vi "#632.vi"() -> (3 "Arguments":string)   [LabVIEW 2017, in "testcase-issue.lvclass"]
uses:
  testcase-issue.lvclass
  src/user.lib/_NEVSTOP/Communicable State Machine(CSM)/Utility/_support/Periodic String Filter Level.ctl
  src/user.lib/_NEVSTOP/Communicable State Machine(CSM)/Utility/Periodic String Filter Setting.ctl
  30fe3c43-9356-4971-8d24-89df9aa8dda5.vi
  src/user.lib/_NEVSTOP/Communicable State Machine(CSM)/_Shared/Change Speed Counter.vi
  src/user.lib/_NEVSTOP/Communicable State Machine(CSM)/_Shared/Debounced Signal.vi
  src/user.lib/_NEVSTOP/Communicable State Machine(CSM)/AdvanceAPI/CSM - Revert Arguments-Safe String.vi
  src/user.lib/_NEVSTOP/Communicable State Machine(CSM)/_Shared/Trim Single-line Text.vi
  src/user.lib/_NEVSTOP/Communicable State Machine(CSM)/AdvanceAPI/CSM - Make String Arguments Safe.vi
  src/user.lib/_NEVSTOP/Communicable State Machine(CSM)/AdvanceAPI/CSM - Break Down Multiple States String.vi
  src/user.lib/_NEVSTOP/Communicable State Machine(CSM)/AdvanceAPI/CSM - Compact Multiple States.vi
  src/user.lib/_NEVSTOP/Communicable State Machine(CSM)/AdvanceAPI/CSM - Keywords.vi
  src/user.lib/_NEVSTOP/Communicable State Machine(CSM)/Communicable State Machine.lvlib
  src/user.lib/_NEVSTOP/Communicable State Machine(CSM)/_Shared/CSM Shared.lvlib
panel:
  out "LogInQ":i32
  out "State History":string
  out "log handling Speed(#/s)":dbl
  out "LogInQ change(#/s)":dbl
  out "Level":T1
  in  "Stop":bool
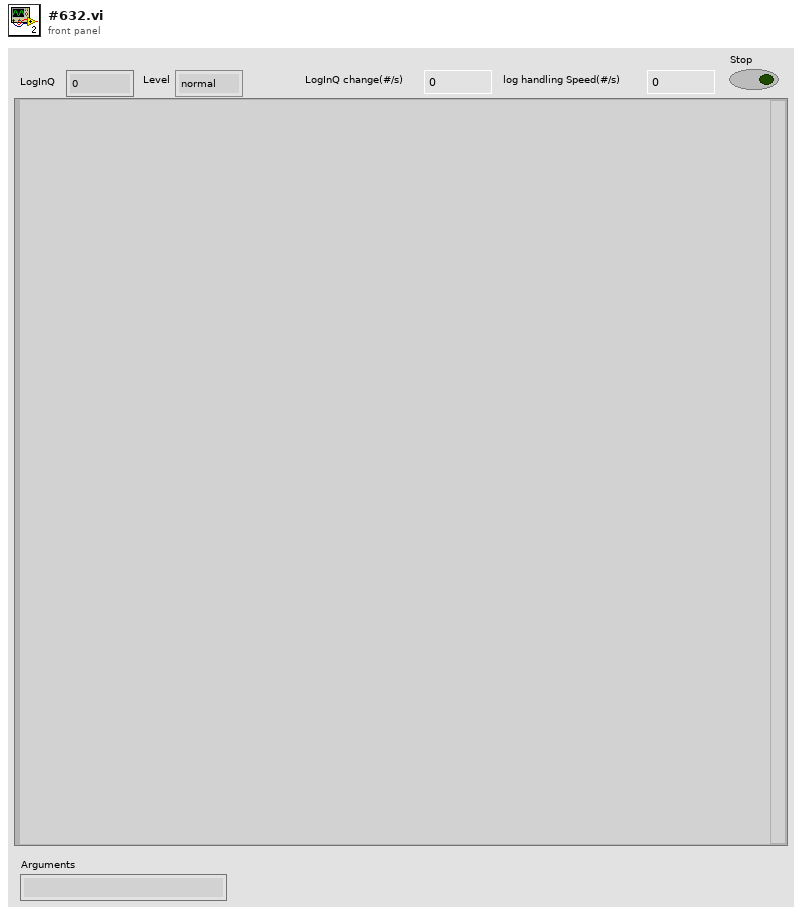
[diagram p1: front panel]
types:
  T1 = typedef "Communicable State Machine.lvlib/Periodic String Filter Level.ctl" = enum16{"normal", "L1", "L2", "L3", "L4"}
  T2 = typedef "Communicable State Machine.lvlib/Periodic String Filter Setting.ctl" = cluster{"threashold(#/s)":dbl, "Check Peroid(s)":dbl}
  T3 = typedef "Communicable State Machine.lvlib/_CSM_GlobalLog_MSG.ctl" = cluster{"Name (\"\" to Use UUID)":string, "Current State":string, "Arguments":string, "Source Message":T4, "Source Module":string, "Complete(T)/Start(F)":bool, "LogType":T5, "Time Stamp":timestamp}
  T4 = typedef "Communicable State Machine.lvlib/_CSM_Response Source Message.ctl" = cluster{"‘State":string, "’Arguments":string, "’Error":errorcluster}
  T5 = typedef "Communicable State Machine.lvlib/_CSM_GlobalLog_MSG_TYPE.ctl" = enum16{"User Log", "State Change", "Status", "Interrupt", "Register", "Unregister", "Error Log", "Module Created", "Module Destroyed", "Async Message", "No-Rep Async Message", "Sync Message", "AsyncMsg Complete", "SyncMsg Complete"}
  T6 = enum32{"Invalid", "Standard", "Closed", "Hidden", "Minimized", "Maximized"}
  T7 = enum32{"invalid app kind", "Development System", "Run Time System", "Student Edition", "Embedded LabVIEW", "Evaluation", "Custom"}
  T8 = cluster{"Current VI Reference":refnum<vi>, "Close Panel on Exit?":bool}
  T9 = cluster{"Core":cluster{"Current VI Reference":refnum<vi>, "Close Panel on Exit?":bool}, "Your Boolean data":bool, "Your string data":string}
  T10 = cluster{"Core":cluster{"Current VI Reference":refnum<vi>, "Close Panel on Exit?":bool}}
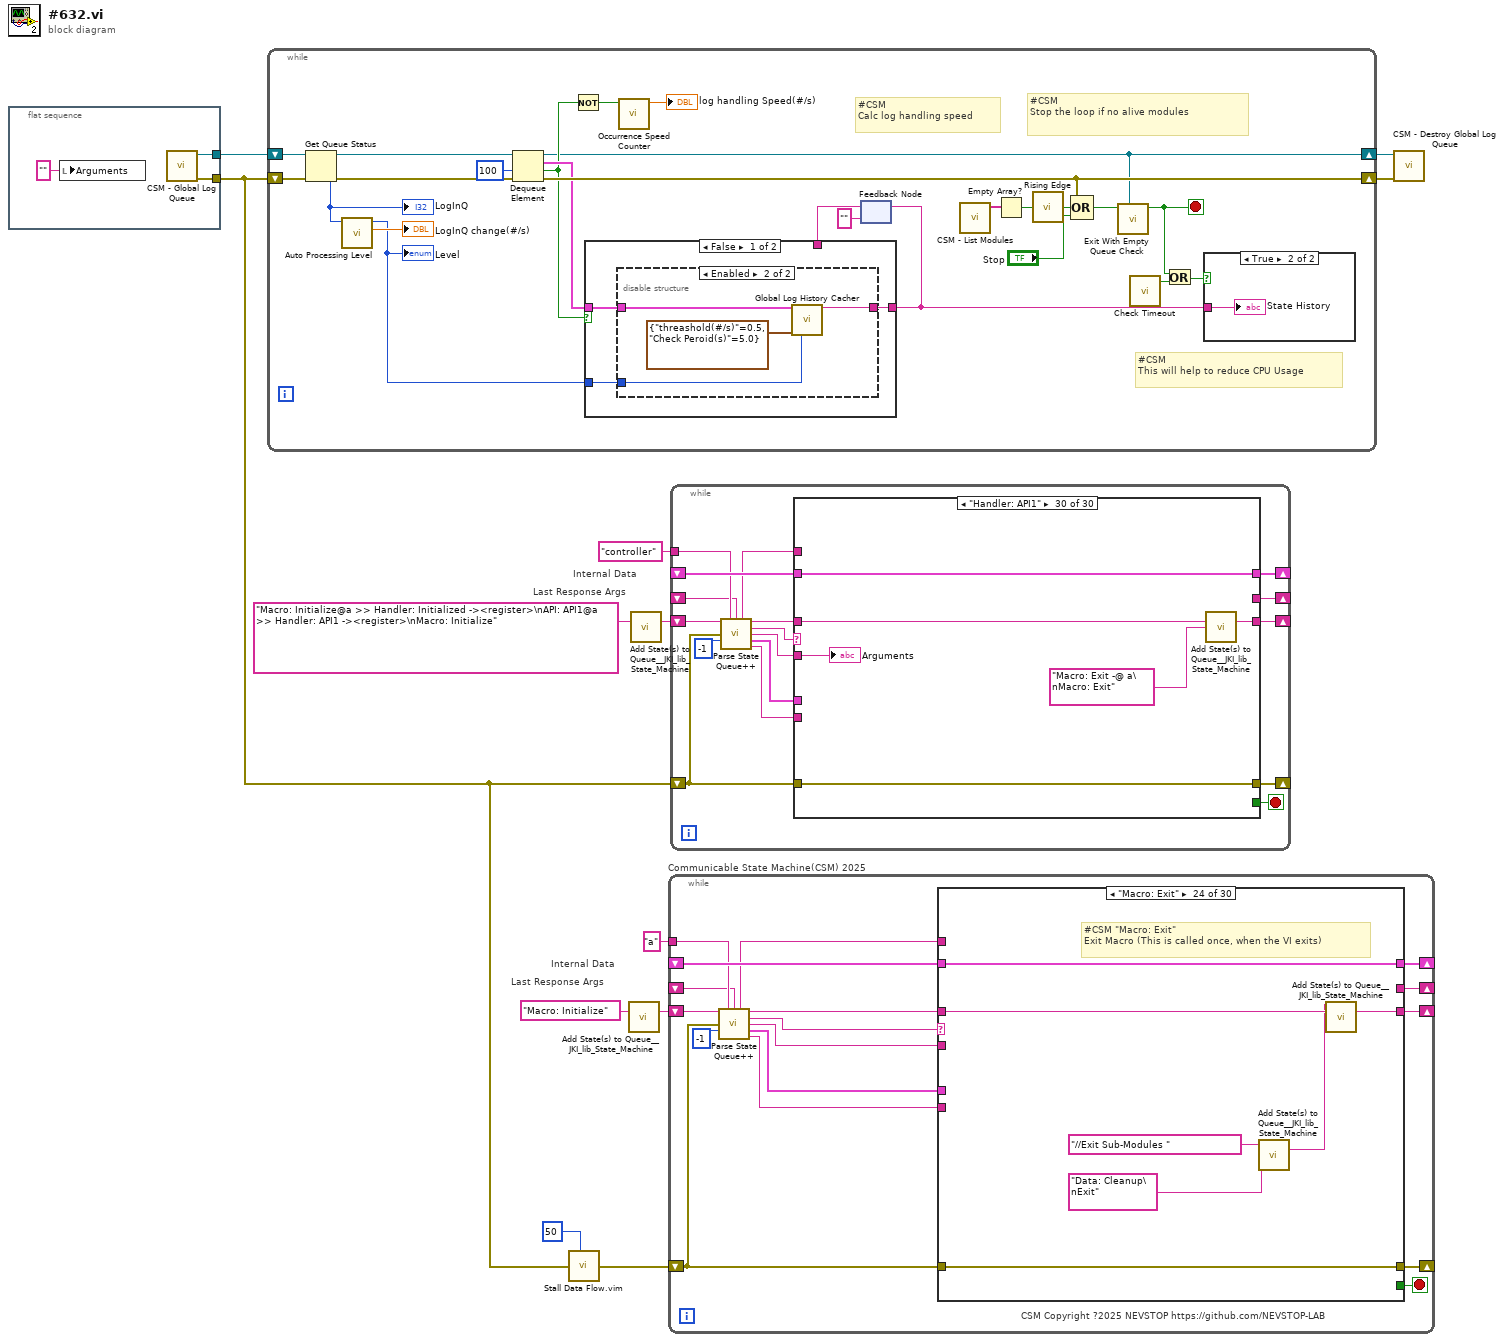
[diagram p0: block diagram]
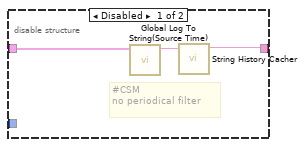
[diagram p2: hidden frame]
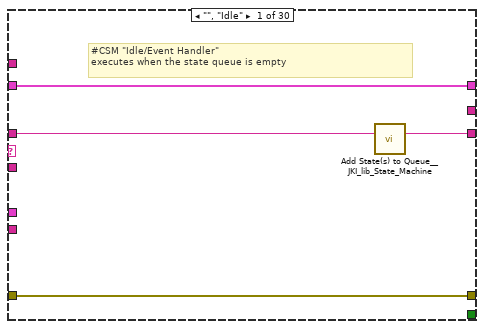
[diagram p5: hidden frame]
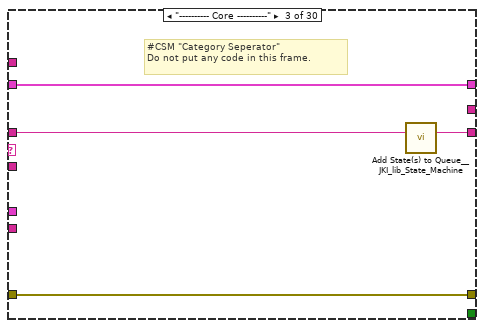
[diagram p7: hidden frame]
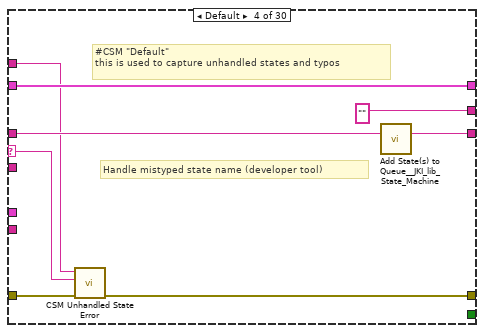
[diagram p8: hidden frame]
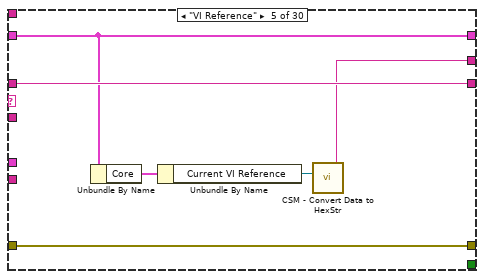
[diagram p9: hidden frame]
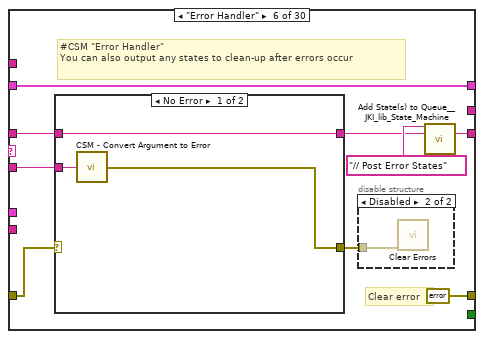
[diagram p10: hidden frame]
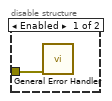
[diagram p11: hidden frame]
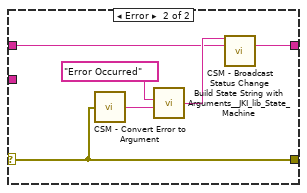
[diagram p12: hidden frame]
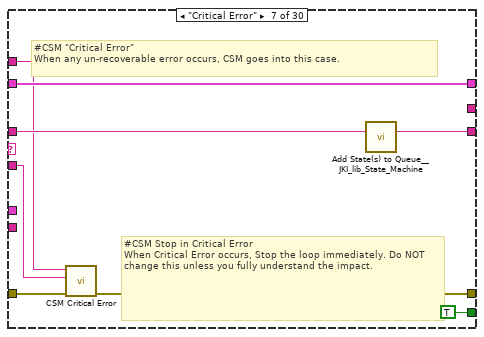
[diagram p13: hidden frame]
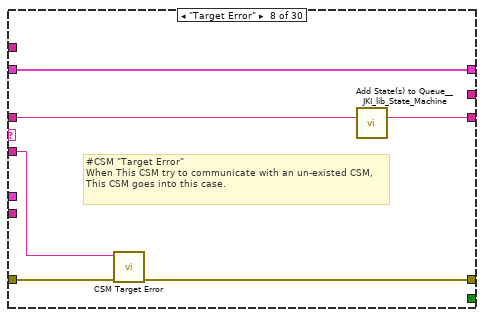
[diagram p14: hidden frame]
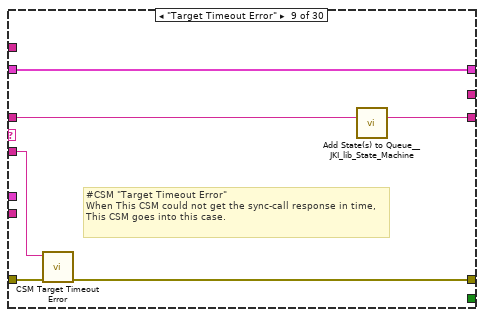
[diagram p15: hidden frame]
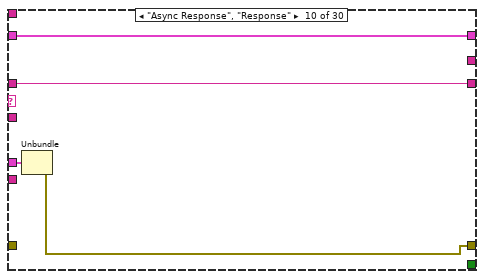
[diagram p16: hidden frame]
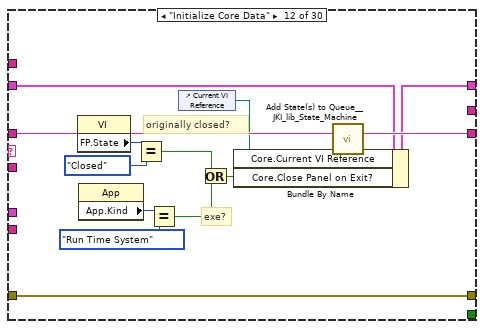
[diagram p18: hidden frame]
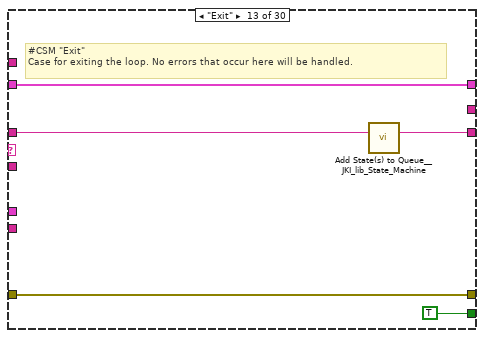
[diagram p19: hidden frame]
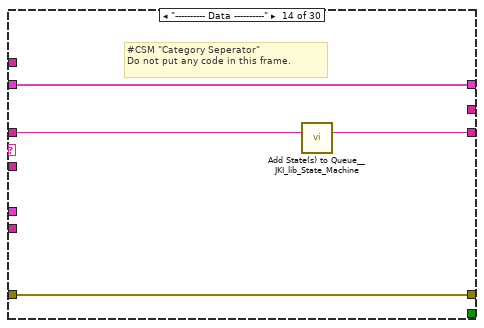
[diagram p20: hidden frame]
diagram:
  # "Last Response Args"
  # "Internal Data"
  # "Last Response Args"
  # "Internal Data"
  n1 = flat-sequence {
    tunnel: [w15] -> w4
    tunnel: [w14] -> w3
    frame #0 {
      n2 = local write "Arguments"("" ("Arguments")) -> ()
      n3 = call "CSM - Global Log Queue.vi"() -> ("error out"=w14:errorcluster, "Global Log Queue"=w15:refnum<queue>)  [unwired: 10 in]
    }
  }
  n4 = while {
    shift-right: [w39] -> w6
    shift-left: w3 -> [w36]
    shift-right: [w23] -> w5
    shift-left: w4 -> [w40]
    stop <- w16 stop-if-true
    # "#CSM\nCalc log handling speed"
    # "#CSM\nStop the loop if no alive modules"
    # "#CSM\nThis will help to reduce CPU Usage"
    n5 = Get Queue Status(queue=w40, error in (no error)=w36) -> (queue out=w38:refnum<queue>, error out=w37:errorcluster, # elements in queue=w19:i32)  [unwired: 1 in, 5 out]
    "LogInQ" <- w19
    n6 = call "Auto Processing Level.vi"("#Left In Q"=w19) -> ("LogInQ Changing Speed (#/s)"=→"LogInQ change(#/s)":dbl, "Level"=w18:T1)  [unwired: 8 in, 1 out]
    "Level" <- w18
    n7 = Dequeue Element(queue=w38, timeout in ms (-1)=100, error in (no error)=w37) -> (queue out=w23:refnum<queue>, element=w35:T3, timed out?=w25:bool, error out=w39:errorcluster)
    n8 = Not(x=w25) -> (.not. x?=w24:bool)
    n9 = call "Occurrence Speed Counter.vi"("Occured? (T)"=w24) -> ("Speed (#/s)"=→"log handling Speed(#/s)":dbl)  [unwired: 8 in, 2 out]
    n10 = feedback #1("" ("String Cache")) -> (w31:string)
    n11 = case shown="False" w25 {
      tunnel: w35 -> [w43 _]
      tunnel: [w42 w51] -> w32
      tunnel: w31 -> [_ w51]
      tunnel: w18 -> [w41 _]
      frame False {
        n12 = disable-structure shown="Enabled" {
          disable-tunnel: w43 -> [w46 w49]
          disable-tunnel: [w44 w50] -> w42
          disable-tunnel: w41 -> [_ w48]
          frame Disabled {
            # "#CSM \nno periodical filter"
            n13 = call "Global Log To String(Source Time).vi"("Log"=w46) -> ("Log String"=w45:string)  [unwired: 9 in]
            n14 = call "String History Cacher.vi"("String"=w45) -> ("String Cache"=w44:string)  [unwired: 10 in]
          }
          frame Enabled {
            n15 = call "Global Log History Cacher.vi"("Global Log Data"=w49, "Settings"=T2 {"threashold(#/s)"=0.5, "Check Peroid(s)"=5.0}, "Level (Normal)"=w48) -> ("String Cache"=w50:string)  [unwired: 12 in]
          }
        }
      }
      frame True {
      }
    }
    n16 = feedback-in #1(w32) -> ()
    n17 = call "CSM - List Modules.vi"() -> ("Module Names"=w30:string[])  [unwired: 10 in, 1 out]
    n18 = Empty Array?(array=w30) -> (empty?=w29:bool)
    n19 = call "Rising Edge.vi"("Signal"=w29) -> ("Rising Edge"=w28:bool)
    n20 = Compound Arithmetic op=OR(w39, w28, "Stop") -> (w21:bool)
    n21 = call "Exit With Empty Queue Check.vi"("Queue"=w23, "Stop"=w21) -> ("Exit"=w16:bool)  [unwired: 8 in, 1 out]
    n22 = call "Check Timeout.vi"() -> ("Timeout"=w33:bool)  [unwired: 8 in]
    n23 = Or(x=w16, y=w33) -> (x .or. y?=w22:bool)
    n24 = case shown="True" w22 {
      tunnel: w32 -> [_ w52]
      frame False {
      }
      frame True {
        "State History" <- w52
      }
    }
  }
  n25 = call "Stall Data Flow.vim"("value in"=w3, "milliseconds to wait"=u32 50) -> ("value out"=w2:errorcluster)  [unwired: 1 out]
  n26 = call <vilib>:"Add State(s) to Queue__JKI_lib_State_Machine.vi"("State(s) in (\"\")"="Macro: Initialize" ("Init State(\"Macro: Initialize\")")) -> ("States Out"=w10:string)  [unwired: 14 in]
  n27 = call <vilib>:"Add State(s) to Queue__JKI_lib_State_Machine.vi"("State(s) in (\"\")"="Macro: Initialize@a >> Handler: Initialized -><register>\nAPI: API1@a >> Handler: API1 -><register>\nMacro: Initialize" ("Init State(\"Macro: Initialize\")")) -> ("States Out"=w9:string)  [unwired: 14 in]
  n28 = while "Communicable State Machine(CSM) 2025" {
    shift-right: [w64] -> _
    shift-left: _ -> [w63]
    shift-right: [w67] -> _
    shift-left: w2 -> [w62]
    shift-right: [w66] -> _
    shift-left: w10 -> [w68]
    tunnel: "a" ("Name (\"\" to Use UUID)") -> [w60]
    shift-right: [w61] -> _
    shift-left: _ -> [w54]
    stop <- w65 stop-if-true
    # "CSM Copyright ?2025 NEVSTOP https://github.com/NEVSTOP-LAB"
    n29 = call "Parse State Queue++.vi"("State Queue"=w68, "Name (\"\" to Use UUID)"=w60, "Response Arguments"=w54, "Previous Error"=w62, "Dequeue (1 ms)"=-1 ("Timeout")) -> ("Name Used"=w55:string, "Remaining States"=w69:string, "Current State"=w59:string, "Arguments"=w58:string, "Additional Information"=w57:T4, "Source CSM"=w56:string)  [unwired: 5 in]
    n30 = case shown="\"Macro: Exit\"" w59 {
      selector: w59 -> [_ _ _ w83 _ _ _ _ _ _ _ _ _ _ _ _ _ _ _ _ _ _ _ _ _ _ _ _ _ _]
      tunnel: w69 -> [w70 w75 w80 w87 w93 w99 w120 w126 w132 w140 w151 w165 w170 w174 w181 w183 w190 w194 w198 w204 w219 w288 w294 w301 w303 w308 w312 w317 w321 w325]
      tunnel: w58 -> [_ _ _ _ _ w98 w116 w125 w130 w139 _ _ _ _ _ _ _ _ _ w199 w213 _ _ _ _ _ _ _ _ _]
      tunnel: w63 -> [w71 w74 w77 w85 w92 w102 w121 w127 w133 w142 w150 w158 w168 w171 _ w182 w185 w191 w196 w202 w215 w285 w291 w298 w302 w307 w311 w314 w318 w322]
      tunnel: [w72 w76 w78 w81 w94 errorcluster {"status"=FALSE, "code"=0, "source"=""} ("error out") w117 w123 w129 w145 w152 w162 w167 w172 w178 w184 w186 w192 w195 w200 w216 w286 w292 w299 w304 w309 w313 w315 w319 w323] -> w67
      tunnel: w62 -> [w72 w76 w78 w88 w94 w100 w122 w124 w131 _ w152 w162 w167 w172 w178 w184 w187 w192 w195 w201 w217 w286 w292 w299 w304 w309 w313 w315 w319 w323]
      tunnel: [w73 w75 w79 w86 w93 w95 w119 w128 w134 w141 w151 w164 w169 w173 w180 w183 w189 w193 w197 w203 w218 w287 w293 w300 w303 w308 w312 w316 w320 w324] -> w66
      tunnel: [_ _ _ _ _ _ TRUE _ _ _ _ _ TRUE _ _ _ _ _ _ _ _ _ _ _ _ _ _ _ _ _] -> w65
      tunnel: [w71 w74 w77 w85 w92 w102 w121 w127 w133 w143 w150 w163 w168 w171 w179 w182 w185 w191 w196 w202 w215 w285 w291 w298 w302 w307 w311 w314 w318 w322] -> w64
      tunnel: w56 -> [_ _ _ _ _ _ _ _ _ w137 _ _ _ _ _ _ _ _ _ _ _ _ _ _ _ _ _ _ _ _]
      tunnel: w57 -> [_ _ _ _ _ _ _ _ _ w144 _ _ _ _ _ _ _ _ _ _ _ _ _ _ _ _ _ _ _ _]
      tunnel: [_ _ _ "" w89 _ _ _ _ _ _ _ _ _ _ _ _ _ _ _ _ _ _ _ _ "Right" "Wrong" ("HEX String (0-9,A-F)") _ _ _] -> w61
      tunnel: w55 -> [_ _ _ w82 _ _ w115 _ _ _ _ _ _ _ _ _ _ _ _ _ _ _ _ _ _ _ _ _ _ _]
      frame "", "Idle" {
        # "#CSM \"Idle/Event Handler\"\nexecutes when the state queue is empty"
        n31 = call <vilib>:"Add State(s) to Queue__JKI_lib_State_Machine.vi"("State(s) in (\"\")"=w70) -> ("States Out"=w73:string)  [unwired: 14 in]
      }
      frame "CSM Documentation" {
        # "#CSM README FIRST\n\nCommunicable State Machine(CSM) is a LabVIEW application framework that builds upon JKI State Machine(JKISM). It follows the pattern of JKISM and extends the keywords to describe message communication between modules, including concepts such as Sync-Message, Async-Message, Subscription/Unsubscription of status - essential elements for creating reusable code modules. For more information, please visit the CSM wiki: https://nevstop-lab.github.io/CSM-Wiki/\n\nFor instructions on JKI State Machine, visit: http://jki.net/state-machine/\nFor information about CSM, visit: https://github.com/NEVSTOP-LAB"
        # "#CSM \"Documentation\"\nCase for holding CSM Documenation"
      }
      frame "---------- Core ----------" {
        # "#CSM \"Category Seperator\"\nDo not put any code in this frame."
        n32 = call <vilib>:"Add State(s) to Queue__JKI_lib_State_Machine.vi"("State(s) in (\"\")"=w80) -> ("States Out"=w79:string)  [unwired: 14 in]
      }
      frame Default {
        # "#CSM \"Default\"\nthis is used to capture unhandled states and typos"
        # "Handle mistyped state name (developer tool)"
        n33 = call "CSM Unhandled State Error.vi"("error in (no error)"=w88, "Undefined State"=w83, "CSM Name"=w82) -> ("error out"=w81:errorcluster)  [unwired: 8 in]
        n34 = call <vilib>:"Add State(s) to Queue__JKI_lib_State_Machine.vi"("State(s) in (\"\")"=w87) -> ("States Out"=w86:string)  [unwired: 14 in]
      }
      frame "VI Reference" {
        n35 = Unbundle By Name(w92) -> ("Core"=w91:T8)
        n36 = Unbundle By Name(w91) -> ("Current VI Reference"=w90:refnum<vi>)
        n37 = call "CSM - Convert Data to HexStr.vi"("Variant"=w90) -> ("HEX String (0-9,A-F)"=w89:string)  [unwired: 8 in]
      }
      frame "Error Handler" {
        # "#CSM Disable this error dialog if you need"
        # "#CSM \"Error Handler\"\nYou can also output any states to clean-up after errors occur"
        # "Clear error"
        n38 = case shown="No Error" w100 {
          selector: w100 -> [_ w109]
          tunnel: [w108 w111] -> w96
          tunnel: w99 -> [w108 w110]
          tunnel: w98 -> [w107 _]
          tunnel: [w106 w109] -> w101
          frame No Error {
            n39 = call "CSM - Convert Argument to Error.vi"("Argument"=w107) -> ("Error"=w106:errorcluster)  [unwired: 4 in]
            n40 = flat-sequence {
              frame #0 {
                # "#CSM External Error Handler Case\nUsually, it's because This CSM register others' \"Error Occurred\" status with \"Error Handler\". If other CSM have any error, the error will be passed here for central handling."
              }
            }
          }
          frame Error {
            # "#CSM Internal Error Handler Case \nIf any error Occurred, \"Error Occurred\" \nstatus update will be broadcasted to system.\nParameter is Error Cluster."
            n41 = call "CSM - Convert Error to Argument.vi"("Error"=w109) -> ("Argument"=w113:string)  [unwired: 4 in]
            n42 = call <vilib>:"Build State String with Arguments__JKI_lib_State_Machine.vi"("Arguments (\"\")"=w113, "State"="Error Occurred" ("Status with Arguments")) -> ("State with Arguments"=w112:string)  [unwired: 4 in]
            n43 = call "CSM - Broadcast Status Change.vi"("Status With Arguments"=w112, "State Queue"=w110) -> ("Remaining States"=w111:string)  [unwired: 13 in]
          }
        }
        n44 = disable-structure shown="Disabled" {
          disable-tunnel: w101 -> [w104 w105]
          frame Enabled {
            n45 = call <vilib>:"General Error Handler.vi"("error in (no error)"=w104) -> ()  [unwired: 10 in, 5 out]
          }
          frame Disabled {
            n46 = call <vilib>:"Clear Errors.vi"("error in (no error)"=w105) -> ()  [unwired: 5 in, 2 out]
          }
        }
        n47 = call <vilib>:"Add State(s) to Queue__JKI_lib_State_Machine.vi"("State(s) in Front (\"\")"="// Post Error States", "State(s) in (\"\")"=w96) -> ("States Out"=w95:string)  [unwired: 13 in]
      }
      frame "Critical Error" {
        # "#CSM Stop in Critical Error\nWhen Critical Error occurs, Stop the loop immediately. Do NOT change this unless you fully understand the impact."
        # "#CSM \"Critical Error\"\nWhen any un-recoverable error occurs, CSM goes into this case."
        n48 = call "CSM Critical Error.vi"("error in (no error)"=w122, "Arugments (As Reason)"=w116, "CSM Name"=w115) -> ("error out"=w117:errorcluster)  [unwired: 8 in]
        n49 = call <vilib>:"Add State(s) to Queue__JKI_lib_State_Machine.vi"("State(s) in (\"\")"=w120) -> ("States Out"=w119:string)  [unwired: 14 in]
      }
      frame "Target Error" {
        # "#CSM \"Target Error\"\nWhen This CSM try to communicate with an un-existed CSM, This CSM goes into this case."
        n50 = call "CSM Target Error.vi"("error in (no error)"=w124, "Arguments (As CSM Name)"=w125) -> ("error out"=w123:errorcluster)  [unwired: 9 in]
        n51 = call <vilib>:"Add State(s) to Queue__JKI_lib_State_Machine.vi"("State(s) in (\"\")"=w126) -> ("States Out"=w128:string)  [unwired: 14 in]
      }
      frame "Target Timeout Error" {
        # "#CSM \"Target Timeout Error\"\nWhen This CSM could not get the sync-call response in time, This CSM goes into this case."
        n52 = call "CSM Target Timeout Error.vi"("error in (no error)"=w131, "Arguments (As CSM Name)"=w130) -> ("error out"=w129:errorcluster)  [unwired: 9 in]
        n53 = call <vilib>:"Add State(s) to Queue__JKI_lib_State_Machine.vi"("State(s) in (\"\")"=w132) -> ("States Out"=w134:string)  [unwired: 14 in]
      }
      frame "Async Response", "Response" {
        n54 = Unbundle(w144) -> ("‘State"=w138:string, "’Arguments"=w136:string, "’Error"=w135:errorcluster)
        n55 = case shown="Default" w138 {
          tunnel: [w149] -> w145
          tunnel: w135 -> [w149]
          tunnel: [w148] -> w143
          tunnel: w142 -> [w148]
          tunnel: [w146] -> w141
          tunnel: w140 -> [w147]
          tunnel: w139 -> [_]
          tunnel: w137 -> [_]
          tunnel: w136 -> [_]
          frame Default {
            # "#CSM Response Comments\nAfter Message is executed, CSM goes to this state for receive the response.\n    For Async Message(->), \"Async Response\" is used. This CSM will goes to \"Async Message Posted\" immediately and receive the \"Async Response\" after the callee finishes the message.\n    For Sync Message(@),  This CSM will wait until the message is done and immediately goes to \"Response\""
            # "#CSM \"Async Response\"\nHandle Async-call Response (\"Async Response\" for ->)"
            # "#CSM \"Response\"\nHandle Sync-call Response (\"Response\" for -@)"
            n56 = call <vilib>:"Add State(s) to Queue__JKI_lib_State_Machine.vi"("State(s) in (\"\")"=w147) -> ("States Out"=w146:string)  [unwired: 14 in]
          }
        }
      }
      frame "Async Message Posted" {
        # "#CSM \"Async Message Posted\"\nAfter Async Message is posted (-> or ->| ), CSM goes to this state for post-action.\nYou can use Argument - State to tell which Async Message is called."
      }
      frame "Initialize Core Data" {
        # "#CSM \"Initialize Core Data\"\nThis is used to determine panel behavior on exit"
        # "originally closed?"
        # "exe?"
        # "If panel starts closed or is an EXE, then close it when we exit"
        n57 = property class="VI"() -> ("FP.State"=w155:T6)  [unwired: 2 in, 2 out]
        n58 = property class="App"() -> ("App.Kind"=w161:T7)  [unwired: 2 in, 2 out]
        n59 = control-ref of="Current VI Reference"() -> (w156:refnum<vi>)
        n60 = Equal?(x=w155, y=T6."Closed" ("Front Panel Window:State")) -> (x = y?=w153:bool)
        n61 = Equal?(x=w161, y=T7."Run Time System" ("Application:Kind")) -> (x = y?=w159:bool)
        n62 = Or(x=w153, y=w159) -> (x .or. y?=w157:bool)
        n63 = Bundle By Name(cluster=w158, "Core.Current VI Reference"=w156, "Core.Close Panel on Exit?"=w157) -> (w163:T9)
        n64 = call <vilib>:"Add State(s) to Queue__JKI_lib_State_Machine.vi"("State(s) in (\"\")"=w165) -> ("States Out"=w164:string)  [unwired: 14 in]
      }
      frame "Exit" {
        # "#CSM \"Exit\"\nCase for exiting the loop. No errors that occur here will be handled."
        n65 = call <vilib>:"Add State(s) to Queue__JKI_lib_State_Machine.vi"("State(s) in (\"\")"=w170) -> ("States Out"=w169:string)  [unwired: 14 in]
      }
      frame "---------- Data ----------" {
        # "#CSM \"Category Seperator\"\nDo not put any code in this frame."
        n66 = call <vilib>:"Add State(s) to Queue__JKI_lib_State_Machine.vi"("State(s) in (\"\")"=w174) -> ("States Out"=w173:string)  [unwired: 14 in]
      }
      frame "Data: Initialize" {
        w175 = T8 {"Current VI Reference"=refnum, "Close Panel on Exit?"=FALSE}  # Core
        w177 = TRUE  # Your Boolean data
        w176 = ""  # Your string data
        # "#CSM do not delete - used by framework"
        # "#CSM Expand Bundle to add new data elements to shift register data."
        # "#CSM Add new data here."
        # "Initialize the shift-register data, here.\n(data names are defined by what you wire into the bundle function)"
        n67 = Bundle("Core"=w175, "Your Boolean data"=w177, "Your string data"=w176) -> (w179:T9)  [unwired: 1 in]
        n68 = call <vilib>:"Add State(s) to Queue__JKI_lib_State_Machine.vi"("State(s) in (\"\")"=w181) -> ("States Out"=w180:string)  [unwired: 14 in]
      }
      frame "Data: Update Indicators" {
      }
      frame "Data: Cleanup" {
        # "Cleanup any data and references, here.\n(this is called automatically, by the Macro: Exit)"
        n69 = Unbundle By Name(w185) -> ("Core.Current VI Reference"=w188:refnum<vi>)
        n70 = Close Reference(reference=w188, error in (no error)=w187) -> (error out=w186:errorcluster)
        n71 = call <vilib>:"Add State(s) to Queue__JKI_lib_State_Machine.vi"("State(s) in (\"\")"=w190) -> ("States Out"=w189:string)  [unwired: 14 in]
      }
      frame "---------- UI ----------" {
        # "#CSM \"Category Seperator\"\nDo not put any code in this frame."
        n72 = call <vilib>:"Add State(s) to Queue__JKI_lib_State_Machine.vi"("State(s) in (\"\")"=w194) -> ("States Out"=w193:string)  [unwired: 14 in]
      }
      frame "UI: Initialize" {
        # "#CSM \"UI: Initialize\"\nInitialize the User Interface, here.\n(this is called automatically, by the Macro: Init)"
        n73 = call <vilib>:"Add State(s) to Queue__JKI_lib_State_Machine.vi"("State(s) in (\"\")"=w198) -> ("States Out"=w197:string)  [unwired: 14 in]
      }
      frame "UI: Cursor Set" {
        # "#CSM \"UI: Cursor Set\"\nSet and Unset Cursor Busy.\n(Usage: \"UI: Cursor Set >> Busy|Idle\")"
        # "Argument"
        n74 = disable-structure shown="TARGET_TYPE!=Windows" {
          disable-tunnel: w201 -> [w207 w212]
          disable-tunnel: [w206 w212] -> w200
          disable-tunnel: w199 -> [w205 _]
          frame condition #0 (active) {
            n75 = case shown="\"Idle\", Default" w205 {
              tunnel: w207 -> [w209 w211]
              tunnel: [w208 w210] -> w206
              frame "Idle", Default {
                n76 = call <vilib>:"Unset Busy.vi"("error in (no error)"=w209) -> ("error out"=w208:errorcluster)  [unwired: 10 in]
              }
              frame "Busy" {
                n77 = call <vilib>:"Set Busy.vi"("error in (no error)"=w211) -> ("error out"=w210:errorcluster)  [unwired: 9 in, 1 out]
              }
            }
          }
          frame condition #1 {
          }
        }
        n78 = call <vilib>:"Add State(s) to Queue__JKI_lib_State_Machine.vi"("State(s) in (\"\")"=w204) -> ("States Out"=w203:string)  [unwired: 14 in]
      }
      frame "UI: Front Panel State" {
        # "#CSM \"UI: Front Panel State\"\nSet Front Panel Open or Closed\n(Usage: \"UI: Front Panel State >> Open|Close\")"
        # "Argument"
        n79 = Unbundle By Name(w215) -> ("Core.Current VI Reference"=w214:refnum<vi>)
        n80 = call <vilib>:"Add State(s) to Queue__JKI_lib_State_Machine.vi"("State(s) in (\"\")"=w219) -> ("States Out"=w218:string)  [unwired: 14 in]
        n81 = case shown="\"Close\", \"Closed\"" w213 {
          tunnel: w217 -> [w225 w240 w251 w264 w277]
          tunnel: [w227 w241 w253 w266 w279] -> w216
          tunnel: w214 -> [w226 w238 w252 w265 w278]
          frame "Open", "Standard", Default {
            w220 = T6."Standard" ("State")
            n82 = property class="VI"(reference=w226, error in=w225) -> (reference out=w223:refnum<vi>, error out=w224:errorcluster, "FP.State"=w222:T6)
            n83 = Not Equal?(x=w222, y=w220) -> (x != y?=w221:bool)
            n84 = case shown="True" w221 {
              tunnel: [w231 w233] -> w227
              tunnel: w224 -> [w230 w233]
              tunnel: w223 -> [w229 _]
              tunnel: w220 -> [w228 _]
              frame True {
                n85 = invoke class="VI" method="FP.Open"(reference=w229, error in=w230, "Activate"=TRUE, "State"=w228) -> (error out=w231:errorcluster)  [unwired: 1 in, 4 out]
              }
              frame False {
              }
            }
          }
          frame "Close", "Closed" {
            n86 = property class="VI"(reference=w238, error in=w240) -> (reference out=w237:refnum<vi>, error out=w239:errorcluster, "FP.State"=w235:T6)
            n87 = Not Equal?(x=w235, y=T6."Closed" ("Front Panel Window:State")) -> (x != y?=w234:bool)
            n88 = case shown="False" w234 {
              tunnel: [w242 w245] -> w241
              tunnel: w239 -> [w242 w244]
              tunnel: w237 -> [_ w243]
              frame False {
              }
              frame True {
                n89 = invoke class="VI" method="FP.Close"(reference=w243, error in=w244) -> (error out=w245:errorcluster)  [unwired: 1 in, 2 out]
              }
            }
          }
          frame "Hidden", "Hide" {
            w246 = T6."Hidden" ("State")
            n90 = property class="VI"(reference=w252, error in=w251) -> (reference out=w249:refnum<vi>, error out=w250:errorcluster, "FP.State"=w248:T6)
            n91 = Not Equal?(x=w248, y=w246) -> (x != y?=w247:bool)
            n92 = case shown="True" w247 {
              tunnel: [w257 w258] -> w253
              tunnel: w250 -> [w256 w258]
              tunnel: w249 -> [w255 _]
              tunnel: w246 -> [w254 _]
              frame True {
                n93 = invoke class="VI" method="FP.Open"(reference=w255, error in=w256, "State"=w254) -> (error out=w257:errorcluster)  [unwired: 2 in, 4 out]
              }
              frame False {
              }
            }
          }
          frame "Minimize", "Minimized" {
            w259 = T6."Minimized" ("State")
            n94 = property class="VI"(reference=w265, error in=w264) -> (reference out=w262:refnum<vi>, error out=w263:errorcluster, "FP.State"=w261:T6)
            n95 = Not Equal?(x=w261, y=w259) -> (x != y?=w260:bool)
            n96 = case shown="True" w260 {
              tunnel: [w270 w271] -> w266
              tunnel: w263 -> [w269 w271]
              tunnel: w262 -> [w268 _]
              tunnel: w259 -> [w267 _]
              frame True {
                n97 = invoke class="VI" method="FP.Open"(reference=w268, error in=w269, "State"=w267) -> (error out=w270:errorcluster)  [unwired: 2 in, 4 out]
              }
              frame False {
              }
            }
          }
          frame "Maximize", "Maximized" {
            w272 = T6."Maximized" ("State")
            n98 = property class="VI"(reference=w278, error in=w277) -> (reference out=w275:refnum<vi>, error out=w276:errorcluster, "FP.State"=w274:T6)
            n99 = Not Equal?(x=w274, y=w272) -> (x != y?=w273:bool)
            n100 = case shown="True" w273 {
              tunnel: [w283 w284] -> w279
              tunnel: w276 -> [w282 w284]
              tunnel: w275 -> [w281 _]
              tunnel: w272 -> [w280 _]
              frame True {
                n101 = invoke class="VI" method="FP.Open"(reference=w281, error in=w282, "State"=w280) -> (error out=w283:errorcluster)  [unwired: 2 in, 4 out]
              }
              frame False {
              }
            }
          }
        }
      }
      frame "---------- Macro ----------" {
        # "#CSM \"Category Seperator\"\nDo not put any code in this frame."
        n102 = call <vilib>:"Add State(s) to Queue__JKI_lib_State_Machine.vi"("State(s) in (\"\")"=w288) -> ("States Out"=w287:string)  [unwired: 14 in]
      }
      frame "Macro: Initialize" {
        # "#CSM \"Macro: Initialize\"\nInitialization Macro (This is called once, when the VI starts)"
        n103 = call <vilib>:"Add State(s) to Queue__JKI_lib_State_Machine.vi"("State(s) in Front (\"\")"="Data: Initialize\nInitialize Core Data\nData: Update Indicators", "State(s) in (\"\")"=w294, "State(s) at Back (\"\")"="API: API1") -> ("States Out"=w293:string)  [unwired: 12 in]
      }
      frame "Macro: Exit" {
        # "#CSM \"Macro: Exit\"\nExit Macro (This is called once, when the VI exits)"
        n104 = call <vilib>:"Add State(s) to Queue__JKI_lib_State_Machine.vi"("State(s) in Front (\"\")"="//Exit Sub-Modules ", "State(s) at Back (\"\")"="Data: Cleanup\nExit") -> ("States Out"=w296:string)  [unwired: 13 in]
        n105 = call <vilib>:"Add State(s) to Queue__JKI_lib_State_Machine.vi"("State(s) in Front (\"\")"=w296, "State(s) in (\"\")"=w301) -> ("States Out"=w300:string)  [unwired: 13 in]
      }
      frame "---------- API ----------" {
        # "#CSM \"Category Seperator\"\nDo not put any code in this frame."
      }
      frame "API: API1" {
        # "#CSM API Example\nCopy/Rename this case for your own API"
        n106 = Wait (ms)(milliseconds to wait=u32 2000) -> ()  [unwired: 1 out]
      }
      frame "API: API2" {
        # "#CSM API Example\nCopy/Rename this case for your own API"
      }
      frame "---------- Action ----------" {
        # "#CSM \"Category Seperator\"\nDo not put any code in this frame."
        n107 = call <vilib>:"Add State(s) to Queue__JKI_lib_State_Machine.vi"("State(s) in (\"\")"=w317) -> ("States Out"=w316:string)  [unwired: 14 in]
      }
      frame "Action: action1" {
        # "#CSM \"Internal State\"\nThis category is used for holding internal states"
        n108 = call <vilib>:"Add State(s) to Queue__JKI_lib_State_Machine.vi"("State(s) in (\"\")"=w321) -> ("States Out"=w320:string)  [unwired: 14 in]
      }
      frame "Action: action2" {
        # "#CSM \"Internal State\"\nThis category is used for holding internal states"
        n109 = call <vilib>:"Add State(s) to Queue__JKI_lib_State_Machine.vi"("State(s) in (\"\")"=w325) -> ("States Out"=w324:string)  [unwired: 14 in]
      }
    }
  }
  n110 = while {
    shift-right: [w337] -> _
    shift-left: _ -> [w336]
    shift-right: [w340] -> _
    shift-left: w3 -> [w335]
    shift-right: [w339] -> _
    shift-left: w9 -> [w341]
    tunnel: "controller" ("Name (\"\" to Use UUID)") -> [w333]
    shift-right: [w334] -> _
    shift-left: _ -> [w327]
    stop <- w338 stop-if-true
    n111 = call "Parse State Queue++.vi"("State Queue"=w341, "Name (\"\" to Use UUID)"=w333, "Response Arguments"=w327, "Previous Error"=w335, "Dequeue (1 ms)"=-1 ("Timeout")) -> ("Name Used"=w328:string, "Remaining States"=w342:string, "Current State"=w332:string, "Arguments"=w331:string, "Additional Information"=w330:T4, "Source CSM"=w329:string)  [unwired: 5 in]
    n112 = case shown="\"Handler: API1\"" w332 {
      selector: w332 -> [_ _ _ w356 _ _ _ _ _ _ _ _ _ _ _ _ _ _ _ _ _ _ _ _ _ _ _ _ _ _]
      tunnel: w342 -> [w343 w348 w353 w360 w366 w372 w393 w399 w405 w409 w413 w427 w432 w436 w441 w443 w450 w454 w458 w464 w479 w548 w553 w560 w562 w567 w571 w576 w583 w589]
      tunnel: w331 -> [_ _ _ _ _ w371 w389 w398 w403 _ _ _ _ _ _ _ _ _ _ w459 w473 _ _ _ _ _ _ _ _ w584]
      tunnel: w336 -> [w344 w347 w350 w358 w365 w375 w394 w400 w406 w410 w412 w420 w430 w433 _ w442 w445 w451 w456 w462 w475 w545 w550 w557 w561 w566 w570 w573 w581 w586]
      tunnel: [w345 w349 w351 w354 w367 errorcluster {"status"=FALSE, "code"=0, "source"=""} ("error out") w390 w396 w402 w408 w414 w424 w429 w434 w438 w444 w446 w452 w455 w460 w476 w546 w551 w558 w563 w568 w572 w574 w578 w587] -> w340
      tunnel: w335 -> [w345 w349 w351 w361 w367 w373 w395 w397 w404 _ w414 w424 w429 w434 w438 w444 w447 w452 w455 w461 w477 w546 w551 w558 w563 w568 w572 w574 _ w587]
      tunnel: [w346 w348 w352 w359 w366 w368 w392 w401 w407 w409 w413 w426 w431 w435 w440 w443 w449 w453 w457 w463 w478 w547 w552 w559 w562 w567 w571 w575 w582 w588] -> w339
      tunnel: [_ _ _ _ _ _ TRUE _ _ _ _ _ TRUE _ _ _ _ _ _ _ _ _ _ _ _ _ _ _ _ _] -> w338
      tunnel: [w344 w347 w350 w358 w365 w375 w394 w400 w406 w410 w412 w425 w430 w433 w439 w442 w445 w451 w456 w462 w475 w545 w550 w557 w561 w566 w570 w573 w581 w586] -> w337
      tunnel: w329 -> [_ _ _ _ _ _ _ _ _ _ _ _ _ _ _ _ _ _ _ _ _ _ _ _ _ _ _ _ _ _]
      tunnel: w330 -> [_ _ _ _ _ _ _ _ _ w411 _ _ _ _ _ _ _ _ _ _ _ _ _ _ _ _ _ _ _ _]
      tunnel: [_ _ _ "" w362 _ _ _ _ _ _ _ _ _ _ _ _ _ _ _ _ _ _ _ _ "Right" "Wrong" ("HEX String (0-9,A-F)") _ _ _] -> w334
      tunnel: w328 -> [_ _ _ w355 _ _ w388 _ _ _ _ _ _ _ _ _ _ _ _ _ _ _ _ _ _ _ _ _ w580 _]
      frame "", "Idle" {
        # "#CSM \"Idle/Event Handler\"\nexecutes when the state queue is empty"
        n113 = call <vilib>:"Add State(s) to Queue__JKI_lib_State_Machine.vi"("State(s) in (\"\")"=w343) -> ("States Out"=w346:string)  [unwired: 14 in]
      }
      frame "CSM Documentation" {
        # "#CSM \"Documentation\"\nCase for holding CSM Documenation"
      }
      frame "---------- Core ----------" {
        # "#CSM \"Category Seperator\"\nDo not put any code in this frame."
        n114 = call <vilib>:"Add State(s) to Queue__JKI_lib_State_Machine.vi"("State(s) in (\"\")"=w353) -> ("States Out"=w352:string)  [unwired: 14 in]
      }
      frame Default {
        # "#CSM \"Default\"\nthis is used to capture unhandled states and typos"
        # "Handle mistyped state name (developer tool)"
        n115 = call "CSM Unhandled State Error.vi"("error in (no error)"=w361, "Undefined State"=w356, "CSM Name"=w355) -> ("error out"=w354:errorcluster)  [unwired: 8 in]
        n116 = call <vilib>:"Add State(s) to Queue__JKI_lib_State_Machine.vi"("State(s) in (\"\")"=w360) -> ("States Out"=w359:string)  [unwired: 14 in]
      }
      frame "VI Reference" {
        n117 = Unbundle By Name(w365) -> ("Core"=w364:T8)
        n118 = Unbundle By Name(w364) -> ("Current VI Reference"=w363:refnum<vi>)
        n119 = call "CSM - Convert Data to HexStr.vi"("Variant"=w363) -> ("HEX String (0-9,A-F)"=w362:string)  [unwired: 8 in]
      }
      frame "Error Handler" {
        # "#CSM \"Error Handler\"\nYou can also output any states to clean-up after errors occur"
        # "Clear error"
        n120 = case shown="No Error" w373 {
          selector: w373 -> [_ w382]
          tunnel: [w381 w384] -> w369
          tunnel: w372 -> [w381 w383]
          tunnel: w371 -> [w380 _]
          tunnel: [w379 w382] -> w374
          frame No Error {
            n121 = call "CSM - Convert Argument to Error.vi"("Argument"=w380) -> ("Error"=w379:errorcluster)  [unwired: 4 in]
          }
          frame Error {
            n122 = call "CSM - Convert Error to Argument.vi"("Error"=w382) -> ("Argument"=w386:string)  [unwired: 4 in]
            n123 = call <vilib>:"Build State String with Arguments__JKI_lib_State_Machine.vi"("Arguments (\"\")"=w386, "State"="Error Occurred" ("Status with Arguments")) -> ("State with Arguments"=w385:string)  [unwired: 4 in]
            n124 = call "CSM - Broadcast Status Change.vi"("Status With Arguments"=w385, "State Queue"=w383) -> ("Remaining States"=w384:string)  [unwired: 13 in]
          }
        }
        n125 = disable-structure shown="Disabled" {
          disable-tunnel: w374 -> [w377 w378]
          frame Enabled {
            n126 = call <vilib>:"General Error Handler.vi"("error in (no error)"=w377) -> ()  [unwired: 10 in, 5 out]
          }
          frame Disabled {
            n127 = call <vilib>:"Clear Errors.vi"("error in (no error)"=w378) -> ()  [unwired: 5 in, 2 out]
          }
        }
        n128 = call <vilib>:"Add State(s) to Queue__JKI_lib_State_Machine.vi"("State(s) in Front (\"\")"="// Post Error States", "State(s) in (\"\")"=w369) -> ("States Out"=w368:string)  [unwired: 13 in]
      }
      frame "Critical Error" {
        # "#CSM Stop in Critical Error\nWhen Critical Error occurs, Stop the loop immediately. Do NOT change this unless you fully understand the impact."
        # "#CSM \"Critical Error\"\nWhen any un-recoverable error occurs, CSM goes into this case."
        n129 = call "CSM Critical Error.vi"("error in (no error)"=w395, "Arugments (As Reason)"=w389, "CSM Name"=w388) -> ("error out"=w390:errorcluster)  [unwired: 8 in]
        n130 = call <vilib>:"Add State(s) to Queue__JKI_lib_State_Machine.vi"("State(s) in (\"\")"=w393) -> ("States Out"=w392:string)  [unwired: 14 in]
      }
      frame "Target Error" {
        # "#CSM \"Target Error\"\nWhen This CSM try to communicate with an un-existed CSM, This CSM goes into this case."
        n131 = call "CSM Target Error.vi"("error in (no error)"=w397, "Arguments (As CSM Name)"=w398) -> ("error out"=w396:errorcluster)  [unwired: 9 in]
        n132 = call <vilib>:"Add State(s) to Queue__JKI_lib_State_Machine.vi"("State(s) in (\"\")"=w399) -> ("States Out"=w401:string)  [unwired: 14 in]
      }
      frame "Target Timeout Error" {
        # "#CSM \"Target Timeout Error\"\nWhen This CSM could not get the sync-call response in time, This CSM goes into this case."
        n133 = call "CSM Target Timeout Error.vi"("error in (no error)"=w404, "Arguments (As CSM Name)"=w403) -> ("error out"=w402:errorcluster)  [unwired: 9 in]
        n134 = call <vilib>:"Add State(s) to Queue__JKI_lib_State_Machine.vi"("State(s) in (\"\")"=w405) -> ("States Out"=w407:string)  [unwired: 14 in]
      }
      frame "Async Response", "Response" {
        n135 = Unbundle(w411) -> ("’Error"=w408:errorcluster)  [unwired: 2 out]
      }
      frame "Async Message Posted" {
        # "#CSM \"Async Message Posted\"\nAfter Async Message is posted (-> or ->| ), CSM goes to this state for post-action.\nYou can use Argument - State to tell which Async Message is called."
      }
      frame "Initialize Core Data" {
        # "originally closed?"
        # "exe?"
        n136 = property class="VI"() -> ("FP.State"=w417:T6)  [unwired: 2 in, 2 out]
        n137 = property class="App"() -> ("App.Kind"=w423:T7)  [unwired: 2 in, 2 out]
        n138 = Equal?(x=w417, y=T6."Closed" ("Front Panel Window:State")) -> (x = y?=w415:bool)
        n139 = Equal?(x=w423, y=T7."Run Time System" ("Application:Kind")) -> (x = y?=w421:bool)
        n140 = control-ref of="Current VI Reference"() -> (w418:refnum<vi>)
        n141 = Or(x=w415, y=w421) -> (x .or. y?=w419:bool)
        n142 = Bundle By Name(cluster=w420, "Core.Current VI Reference"=w418, "Core.Close Panel on Exit?"=w419) -> (w425:T10)
        n143 = call <vilib>:"Add State(s) to Queue__JKI_lib_State_Machine.vi"("State(s) in (\"\")"=w427) -> ("States Out"=w426:string)  [unwired: 14 in]
      }
      frame "Exit" {
        # "#CSM \"Exit\"\nCase for exiting the loop. No errors that occur here will be handled."
        n144 = call <vilib>:"Add State(s) to Queue__JKI_lib_State_Machine.vi"("State(s) in (\"\")"=w432) -> ("States Out"=w431:string)  [unwired: 14 in]
      }
      frame "---------- Data ----------" {
        # "#CSM \"Category Seperator\"\nDo not put any code in this frame."
        n145 = call <vilib>:"Add State(s) to Queue__JKI_lib_State_Machine.vi"("State(s) in (\"\")"=w436) -> ("States Out"=w435:string)  [unwired: 14 in]
      }
      frame "Data: Initialize" {
        w437 = T8 {"Current VI Reference"=refnum, "Close Panel on Exit?"=FALSE}  # Core
        # "Initialize the shift-register data, here.\n(data names are defined by what you wire into the bundle function)"
        n146 = Bundle("Core"=w437) -> (w439:T10)  [unwired: 1 in]
        n147 = call <vilib>:"Add State(s) to Queue__JKI_lib_State_Machine.vi"("State(s) in (\"\")"=w441) -> ("States Out"=w440:string)  [unwired: 14 in]
      }
      frame "Data: Update Indicators" {
      }
      frame "Data: Cleanup" {
        # "Cleanup any data and references, here.\n(this is called automatically, by the Macro: Exit)"
        n148 = Unbundle By Name(w445) -> ("Core.Current VI Reference"=w448:refnum<vi>)
        n149 = Close Reference(reference=w448, error in (no error)=w447) -> (error out=w446:errorcluster)
        n150 = call <vilib>:"Add State(s) to Queue__JKI_lib_State_Machine.vi"("State(s) in (\"\")"=w450) -> ("States Out"=w449:string)  [unwired: 14 in]
      }
      frame "---------- UI ----------" {
        # "#CSM \"Category Seperator\"\nDo not put any code in this frame."
        n151 = call <vilib>:"Add State(s) to Queue__JKI_lib_State_Machine.vi"("State(s) in (\"\")"=w454) -> ("States Out"=w453:string)  [unwired: 14 in]
      }
      frame "UI: Initialize" {
        # "#CSM \"UI: Initialize\"\nInitialize the User Interface, here.\n(this is called automatically, by the Macro: Init)"
        n152 = call <vilib>:"Add State(s) to Queue__JKI_lib_State_Machine.vi"("State(s) in (\"\")"=w458) -> ("States Out"=w457:string)  [unwired: 14 in]
      }
      frame "UI: Cursor Set" {
        # "#CSM \"UI: Cursor Set\"\nSet and Unset Cursor Busy.\n(Usage: \"UI: Cursor Set >> Busy|Idle\")"
        # "Argument"
        n153 = disable-structure shown="Default" {
          disable-tunnel: w461 -> [w467 w472]
          disable-tunnel: [w466 w472] -> w460
          disable-tunnel: w459 -> [w465 _]
          frame condition #0 (active) {
            n154 = case shown="\"Idle\", Default" w465 {
              tunnel: w467 -> [w469 w471]
              tunnel: [w468 w470] -> w466
              frame "Idle", Default {
                n155 = call <vilib>:"Unset Busy.vi"("error in (no error)"=w469) -> ("error out"=w468:errorcluster)  [unwired: 10 in]
              }
              frame "Busy" {
                n156 = call <vilib>:"Set Busy.vi"("error in (no error)"=w471) -> ("error out"=w470:errorcluster)  [unwired: 9 in, 1 out]
              }
            }
          }
          frame condition #1 {
          }
        }
        n157 = call <vilib>:"Add State(s) to Queue__JKI_lib_State_Machine.vi"("State(s) in (\"\")"=w464) -> ("States Out"=w463:string)  [unwired: 14 in]
      }
      frame "UI: Front Panel State" {
        # "#CSM \"UI: Front Panel State\"\nSet Front Panel Open or Closed\n(Usage: \"UI: Front Panel State >> Open|Close\")"
        # "Argument"
        n158 = Unbundle By Name(w475) -> ("Core.Current VI Reference"=w474:refnum<vi>)
        n159 = call <vilib>:"Add State(s) to Queue__JKI_lib_State_Machine.vi"("State(s) in (\"\")"=w479) -> ("States Out"=w478:string)  [unwired: 14 in]
        n160 = case shown="\"Close\", \"Closed\"" w473 {
          tunnel: w477 -> [w485 w500 w511 w524 w537]
          tunnel: [w487 w501 w513 w526 w539] -> w476
          tunnel: w474 -> [w486 w498 w512 w525 w538]
          frame "Open", "Standard", Default {
            w480 = T6."Standard" ("State")
            n161 = property class="VI"(reference=w486, error in=w485) -> (reference out=w483:refnum<vi>, error out=w484:errorcluster, "FP.State"=w482:T6)
            n162 = Not Equal?(x=w482, y=w480) -> (x != y?=w481:bool)
            n163 = case shown="True" w481 {
              tunnel: [w491 w493] -> w487
              tunnel: w484 -> [w490 w493]
              tunnel: w483 -> [w489 _]
              tunnel: w480 -> [w488 _]
              frame True {
                n164 = invoke class="VI" method="FP.Open"(reference=w489, error in=w490, "Activate"=TRUE, "State"=w488) -> (error out=w491:errorcluster)  [unwired: 1 in, 4 out]
              }
              frame False {
              }
            }
          }
          frame "Close", "Closed" {
            n165 = property class="VI"(reference=w498, error in=w500) -> (reference out=w497:refnum<vi>, error out=w499:errorcluster, "FP.State"=w495:T6)
            n166 = Not Equal?(x=w495, y=T6."Closed" ("Front Panel Window:State")) -> (x != y?=w494:bool)
            n167 = case shown="False" w494 {
              tunnel: [w502 w505] -> w501
              tunnel: w499 -> [w502 w504]
              tunnel: w497 -> [_ w503]
              frame False {
              }
              frame True {
                n168 = invoke class="VI" method="FP.Close"(reference=w503, error in=w504) -> (error out=w505:errorcluster)  [unwired: 1 in, 2 out]
              }
            }
          }
          frame "Hidden", "Hide" {
            w506 = T6."Hidden" ("State")
            n169 = property class="VI"(reference=w512, error in=w511) -> (reference out=w509:refnum<vi>, error out=w510:errorcluster, "FP.State"=w508:T6)
            n170 = Not Equal?(x=w508, y=w506) -> (x != y?=w507:bool)
            n171 = case shown="True" w507 {
              tunnel: [w517 w518] -> w513
              tunnel: w510 -> [w516 w518]
              tunnel: w509 -> [w515 _]
              tunnel: w506 -> [w514 _]
              frame True {
                n172 = invoke class="VI" method="FP.Open"(reference=w515, error in=w516, "State"=w514) -> (error out=w517:errorcluster)  [unwired: 2 in, 4 out]
              }
              frame False {
              }
            }
          }
          frame "Minimize", "Minimized" {
            w519 = T6."Minimized" ("State")
            n173 = property class="VI"(reference=w525, error in=w524) -> (reference out=w522:refnum<vi>, error out=w523:errorcluster, "FP.State"=w521:T6)
            n174 = Not Equal?(x=w521, y=w519) -> (x != y?=w520:bool)
            n175 = case shown="True" w520 {
              tunnel: [w530 w531] -> w526
              tunnel: w523 -> [w529 w531]
              tunnel: w522 -> [w528 _]
              tunnel: w519 -> [w527 _]
              frame True {
                n176 = invoke class="VI" method="FP.Open"(reference=w528, error in=w529, "State"=w527) -> (error out=w530:errorcluster)  [unwired: 2 in, 4 out]
              }
              frame False {
              }
            }
          }
          frame "Maximize", "Maximized" {
            w532 = T6."Maximized" ("State")
            n177 = property class="VI"(reference=w538, error in=w537) -> (reference out=w535:refnum<vi>, error out=w536:errorcluster, "FP.State"=w534:T6)
            n178 = Not Equal?(x=w534, y=w532) -> (x != y?=w533:bool)
            n179 = case shown="True" w533 {
              tunnel: [w543 w544] -> w539
              tunnel: w536 -> [w542 w544]
              tunnel: w535 -> [w541 _]
              tunnel: w532 -> [w540 _]
              frame True {
                n180 = invoke class="VI" method="FP.Open"(reference=w541, error in=w542, "State"=w540) -> (error out=w543:errorcluster)  [unwired: 2 in, 4 out]
              }
              frame False {
              }
            }
          }
        }
      }
      frame "---------- Macro ----------" {
        # "#CSM \"Category Seperator\"\nDo not put any code in this frame."
        n181 = call <vilib>:"Add State(s) to Queue__JKI_lib_State_Machine.vi"("State(s) in (\"\")"=w548) -> ("States Out"=w547:string)  [unwired: 14 in]
      }
      frame "Macro: Initialize" {
        # "#CSM \"Macro: Initialize\"\nInitialization Macro (This is called once, when the VI starts)"
        n182 = call <vilib>:"Add State(s) to Queue__JKI_lib_State_Machine.vi"("State(s) in Front (\"\")"="Data: Initialize\nInitialize Core Data\nData: Update Indicators", "State(s) in (\"\")"=w553) -> ("States Out"=w552:string)  [unwired: 13 in]
      }
      frame "Macro: Exit" {
        # "#CSM \"Macro: Exit\"\nExit Macro (This is called once, when the VI exits)"
        n183 = call <vilib>:"Add State(s) to Queue__JKI_lib_State_Machine.vi"("State(s) in Front (\"\")"="//Exit Sub-Modules ", "State(s) at Back (\"\")"="Data: Cleanup\nExit") -> ("States Out"=w555:string)  [unwired: 13 in]
        n184 = call <vilib>:"Add State(s) to Queue__JKI_lib_State_Machine.vi"("State(s) in Front (\"\")"=w555, "State(s) in (\"\")"=w560) -> ("States Out"=w559:string)  [unwired: 13 in]
      }
      frame "---------- API ----------" {
        # "#CSM \"Category Seperator\"\nDo not put any code in this frame."
      }
      frame "API: API1" {
        # "#CSM API Example\nCopy/Rename this case for your own API"
        n185 = Wait (ms)(milliseconds to wait=u32 2000) -> ()  [unwired: 1 out]
      }
      frame "API: API2" {
        # "#CSM API Example\nCopy/Rename this case for your own API"
      }
      frame "---------- Action ----------" {
        # "#CSM \"Category Seperator\"\nDo not put any code in this frame."
        n186 = call <vilib>:"Add State(s) to Queue__JKI_lib_State_Machine.vi"("State(s) in (\"\")"=w576) -> ("States Out"=w575:string)  [unwired: 14 in]
      }
      frame "Handler: Initialized" {
        n187 = call "CSM - Send Message and Wait for Reply.vi"("Current Module (\"\" to Generate an ID)"=w580, "Target Module"="a" ("State"), "State"="API: API2") -> ("error out"=w578:errorcluster)  [unwired: 6 in, 2 out]
        n188 = call <vilib>:"Add State(s) to Queue__JKI_lib_State_Machine.vi"("State(s) in (\"\")"=w583) -> ("States Out"=w582:string)  [unwired: 14 in]
      }
      frame "Handler: API1" {
        n189 = call <vilib>:"Add State(s) to Queue__JKI_lib_State_Machine.vi"("State(s) in (\"\")"=w589, "State(s) at Back (\"\")"="Macro: Exit -@ a\nMacro: Exit" ("State(s) at Back (\"\")")) -> ("States Out"=w588:string)  [unwired: 13 in]
        "Arguments" <- w584
      }
    }
  }
  n190 = call "CSM - Destroy Global Log Queue.vi"("Error In"=w6, "Global Log Queue"=w5) -> ()  [unwired: 9 in, 1 out]
